vi "url sub vi.vi"() -> (3 "body 2":string)   [LabVIEW 2019]
uses:
  <vilib>/httpClient/LabVIEWHTTPClient.lvlib
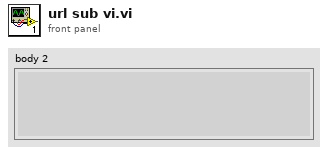
[diagram p1: front panel]
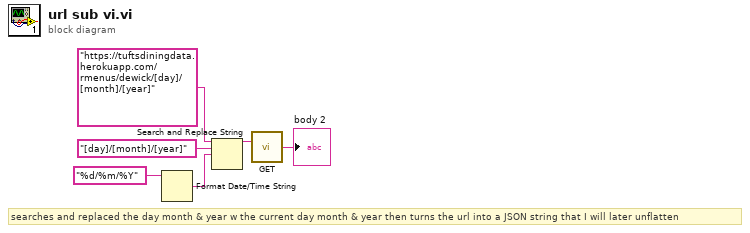
[diagram p0: block diagram]
diagram:
  # "searches and replaced the day month & year w the current day month & year then turns the url into a JSON string that I will later unflatten"
  n1 = Format Date/Time String(time format string (%c)="%d/%m/%Y") -> (date/time string=w4:string)  [unwired: 2 in]
  n2 = Search and Replace String(input string="https://tuftsdiningdata.herokuapp.com/rmenus/dewick/[day]/[month]/[year]" ("url"), search string="[day]/[month]/[year]", replace string=w4) -> (result string=w5:string)  [unwired: 5 in, 3 out]
  n3 = call <vilib>:"GET.vi"("url"=w5) -> ("body"=→"body 2":string)  [unwired: 11 in, 3 out]
